vi "CaLabGet_Main.vi"(0 "PV Name":string[](array[string]), 3 "Field Names":string[](array[string]), 4 "Timeout (3)":u8=3 min=1 step=1, 5 "error in (no error)":errorcluster, 6 "variable PV names (T)":bool=TRUE, 7 "NoMDEL(F)":bool, 9 "Filter":i32) -> (11 "Status":bool, 13 "PV Info":T1[](array[typedef]), 14 "PV Name (dup)":string[](array[string]), 15 "1rst Value (string)":string[](array[string]), 17 "1rst Value (number)":dbl[](array[numeric]), 18 "Value Array (number)":dbl[][](array[numeric]), 19 "error out":errorcluster)   [LabVIEW 2022 SP3, in "CaLab.lvlib"]
doc: "This is a VI for reading values of EPICS variables.\n\nINPUT:\n <b>PV Name(s)</b>\n name array of EPICS variables\n <b>Field Names</b>\n optional\n string array of EPICS fields (\"EGU\", \"DESCRIPTION\" etc.)\n <b>Timeout (3)</b>\n optional\n timeout for Channel Access requests in seconds\n <b>NoMDEL (F)</b>\n optional\n true: ignore monitor dead-band of Channel Access (EPICS)\n <b>variable PV names (T)</b>\n optional\n true: in case of changing PV names at PV name input (performance drop)\n false: in case of constant (array of) PV name(s)\n <b>Error in (no error)</b>\n <b>Filter</b>\n optional\n output filter (this can save ressources and increase performance)\n Following values can be combined with OR:\n PV indicators:\n firstValueAsString = 1\n firstValueAsNumber = 2\n valueArrayAsNumber = 4\n errorOut = 8\n PV Info cluster:\n pviElements = 16\n pviValuesAsString = 32\n pviValuesAsNumber = 64\n pviStatusAsString = 128\n pviStatusAsNumber = 256\n pviSeverityAsString = 512\n pviSeverityAsNumber = 1024\n pviTimestampAsString = 2048\n pviTimestampAsNumber = 4096\n pviFieldNames = 8192\n pviFieldValues = 16384\n pviError = 32768\n\nOUTPUT:\n <b>PV Name</b>\n name array of EPICS variables\n <b>1st Value(string)</b>\n value of variable as String\n shows first item of value array\n <b>1st Value(number)</b>\n value of variable as Double\n shows first item of value array\n <b>Value Array(number)</b>\n all values of variable in Double array\n <b>Error out</b>\n <b>PV Info</b>\n cluster array of full answer\n value array(number)\n PV name\n elements\n size of value array\n value array(string)\n all values of variable in string array\n value array(number)\n elements\n size of value array\n status(string)\n status of EPICS PV as String\n status(number)\n status of EPICS PV as Long\n severity(string)\n severity of EPICS PV as String\n severity(number)\n severity of EPICS PV as Long\n time stamp(string)\n stamp of EPICS PV time as String\n time stamp(number)\n stamp of EPICS PV as Long\n field names\n field values\n string array of requsted EPICS field values\n error IO\n <b>Status</b>\n FALSE: request successful\n TRUE: warnings or errors"
uses:
  CaLab.lvlib
  PV Info.ctl
  <userlib>/calab/lib/calab.dll
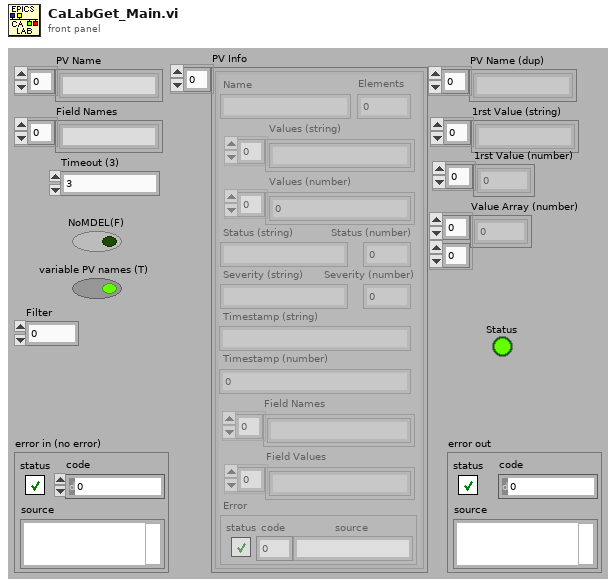
[diagram p1: front panel]
types:
  T1 = typedef "CaLab.lvlib/PV Info.ctl" = cluster{"Name":string, "Elements":i32, "Values (string)":string[], "Values (number)":dbl[], "Status (string)":string, "Status (number)":i16, "Severity (string)":string, "Severity (number)":i16, "Timestamp (string)":string, "Timestamp (number)":i32, "Field Names":string[], "Field Values":string[], "Error":errorcluster}
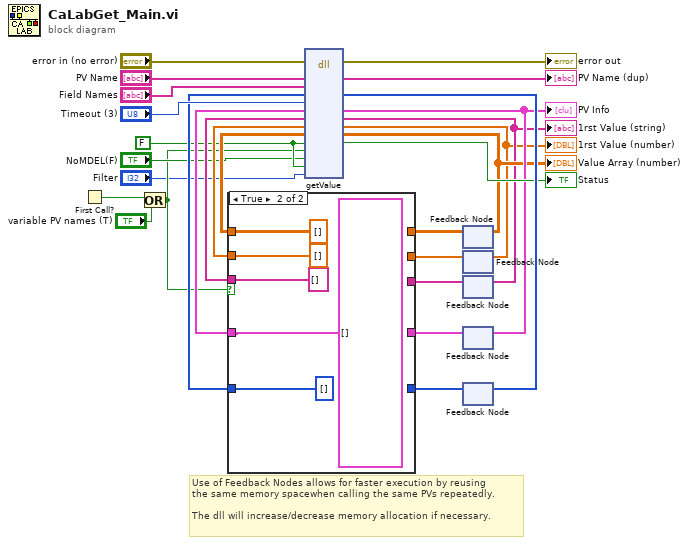
[diagram p0: block diagram]
diagram:
  w6 = FALSE
  # "Use of Feedback Nodes allows for faster execution by reusing\nthe same memory spacewhen calling the same PVs repeatedly.\n\nThe dll will increase/decrease memory allocation if necessary."
  n1 = First Call?() -> (First Call?: T/F=w2:bool)
  n2 = Or(x=w2, y="variable PV names (T)") -> (x .or. y?=w4:bool)
  n3 = feedback #1() -> (w13:dbl[][])  [unwired: 1 out]
  n4 = feedback #2() -> (w11:dbl[])  [unwired: 1 out]
  n5 = feedback #3() -> (w9:string[])  [unwired: 1 out]
  n6 = feedback #4() -> (w23:T1[])  [unwired: 1 out]
  n7 = feedback #5() -> (w22:u64[])  [unwired: 1 out]
  n8 = case shown="True" w4 {
    tunnel: [w33 T1[] [] ("PV Info")] -> w21
    tunnel: [w32 u64[] [] ("value array (number)")] -> w20
    tunnel: w23 -> [w33 _]
    tunnel: w22 -> [w32 _]
    tunnel: [w31 dbl[][] []] -> w15
    tunnel: w13 -> [w31 _]
    tunnel: [w30 dbl[] []] -> w12
    tunnel: w11 -> [w30 _]
    tunnel: [w29 string[] []] -> w10
    tunnel: w9 -> [w29 _]
    frame False {
    }
    frame True {
    }
  }
  n9 = dll-call lib="C:/Program Files/National Instruments/LabVIEW 2023/user.lib/calab/lib/calab.dll" fn="getValue" label="caLabGet"(error in="error in (no error)", "PVNameArray"="PV Name", "FieldNameArray"="Field Names", "IndexArray"=w20, "Timeout"="Timeout (3)", "ResultClusterArray"=w21, "FirstStringValue"=w10, "FirstDoubleValue"=w12, "DoubleValueArray"=w15, "status"=w6, "FirstCall"=w4, "NoMDEL"="NoMDEL(F)", "IsInitialized"=w6, "filter"="Filter") -> (error out=→"error out":errorcluster, "PVNameArray"=→"PV Name (dup)":string[], "IndexArray"=w19:u64[], "ResultClusterArray"=w16:T1[], "FirstStringValue"=w8:string[], "FirstDoubleValue"=w7:dbl[], "DoubleValueArray"=w14:dbl[][], "status"=→"Status":bool)  [unwired: 6 in, 4 out]
  "1rst Value (string)" <- w8
  "1rst Value (number)" <- w7
  "Value Array (number)" <- w14
  "PV Info" <- w16
  n10 = feedback-in #1(w14) -> ()
  n11 = feedback-in #2(w7) -> ()
  n12 = feedback-in #3(w8) -> ()
  n13 = feedback-in #4(w16) -> ()
  n14 = feedback-in #5(w19) -> ()
